vi "NF WF1973_74 sample seq_data.vi"() -> ()   [LabVIEW 2010]
panel:
  in  "Version":dbl=1.0 format="%.2f"
  in  "NEXT?":bool
  in  "Duty 2":dbl=0.01 min=0.01 max=99.99 step=0.01 format="%.2f"
  in  "Phase 2":dbl min=-1800.0 max=1800.0 step=1.0
  in  "Offset 2":dbl min=-10.0 max=10.0 step=1.0 format="%.2f"
  in  "Amplitude 2":dbl min=0.0 max=20.0 step=1.0 format="%.2f"
  in  "Frequency 2":dbl=1e-08 min=1e-08 max=10000000.0 step=0.01 format="%.8f"
  in  "ARB No 2":i16=128
  in  "Duty action 2":u16(ring) items=["Constant", "Keep", "Sweep"]
  in  "Phase action 2":u16(ring) items=["Constant", "Keep", "Sweep"]
  in  "Offset action 2":u16(ring) items=["Constant", "Keep", "Sweep"]
  in  "Amplitude action 2":u16(ring) items=["Constant", "Keep", "Sweep"]
  in  "Frequency action 2":u16(ring) items=["Constant", "Keep", "Sweep"]
  in  "Square Ex(Off) 2":u16(ring) items=["Off", "On"]
  in  "Polarity(Normal) 2":u16(ring) items=["Normal", "Invert"]
  in  "Scale(+/-FS) 2":u16(ring)=1 items=["0/+FS", "+/-FS", "-FS/0"]
  in  "Function(Sin) 2":u16(ring)=2 items=["DC", "Noise", "Sin", "Squ", "USER"]
  in  "Duty":dbl=0.01 min=0.01 max=99.99 step=0.01 format="%.2f"
  in  "Phase":dbl min=-1800.0 max=1800.0 step=1.0
  in  "Offset":dbl min=-10.0 max=10.0 step=1.0 format="%.2f"
  in  "Amplitude":dbl min=0.0 max=20.0 step=1.0 format="%.2f"
  in  "Frequency":dbl=1e-08 min=1e-08 max=10000000.0 step=0.01 format="%.8f"
  in  "ARB No":i16=128
  in  "Duty action":u16(ring) items=["Constant", "Keep", "Sweep"]
  in  "Phase action":u16(ring) items=["Constant", "Keep", "Sweep"]
  in  "Offset action":u16(ring) items=["Constant", "Keep", "Sweep"]
  in  "Amplitude action":u16(ring) items=["Constant", "Keep", "Sweep"]
  in  "Frequency action":u16(ring) items=["Constant", "Keep", "Sweep"]
  in  "Square Ex(Off)":u16(ring) items=["Off", "On"]
  in  "Polarity(Normal)":u16(ring) items=["Normal", "Invert"]
  in  "Scale(+/-FS)":u16(ring)=1 items=["0/+FS", "+/-FS", "-FS/0"]
  in  "Function(Sin)":u16(ring)=2 items=["DC", "Noise", "Sin", "Squ", "USER"]
  in  "Jump count(Infinity)":u16(ring) items=["Infinity", "On"]
  in  "End phase(Off)":u16(ring) items=["Off", "On"]
  in  "Jump step(Off)":u16(ring) items=["Off", "On"]
  in  "Event branch step(Off)":u16(ring) items=["Off", "On"]
  in  "State branch step(Off)":u16(ring) items=["Off", "On"]
  in  "Auto hold(Off)":u16(ring) items=["Off", "On"]
  in  "Parameter(Cont)":u16(ring) items=["Continue", "Stop"]
  in  "End phase":dbl min=0.0 max=360.0 step=1.0
  in  "Jump count":i16=1 min=1 max=999 step=1
  in  "Jump step":i16 min=0 max=255 step=1
  in  "Event branch step":i16 min=0 max=255 step=1
  in  "State branch step":i16 min=0 max=255 step=1
  in  "Step code":i16 min=0 max=15 step=1
  in  "Step time":dbl=0.0001 min=0.0001 max=1000.0 format="%.4f"
  out "Step No":i16
  in  "Trigger polarity(Positive)":u16(ring) items=["Positive", "Negative", "OFF"]
  in  "Digital control(Start)":u16(ring) items=["Start", "State branch"]
  in  "Digital input(Off)":u16(ring) items=["Off", "On"]
  in  "Sync out(Wave)":u16(ring) items=["Wave", "Sequence "]
  in  "Start step(1)":i16=1 min=1 max=255 step=1
  in  "Model(WF1974)":u16(ring)=1 items=["WF1973", "WF1974"]
  out "error out":errorcluster caption="Error OUT"
  in  "error in (no error)":errorcluster caption="Error IN"
  # "Attention!!"
  # "1.Input Model & Version & [Sequence information]\n2.Start VI\n3.Input [Step information] \n4.Input [Channel information] Ch1 & Ch2\n5.Input Parameter\n6.Click to [Next?]\n7.Return to Step 3."
  # "*Firmware version"
  # "This information\n              WF1974 Only!!"
  # "[Ch1 information]"
  # "[Ch2 information]"
  # "[Step information]"
  # "[Sequence information]"
  # "Parameter is \nCont>Next step\nStop>End"
  # "End"
  # "Next step"
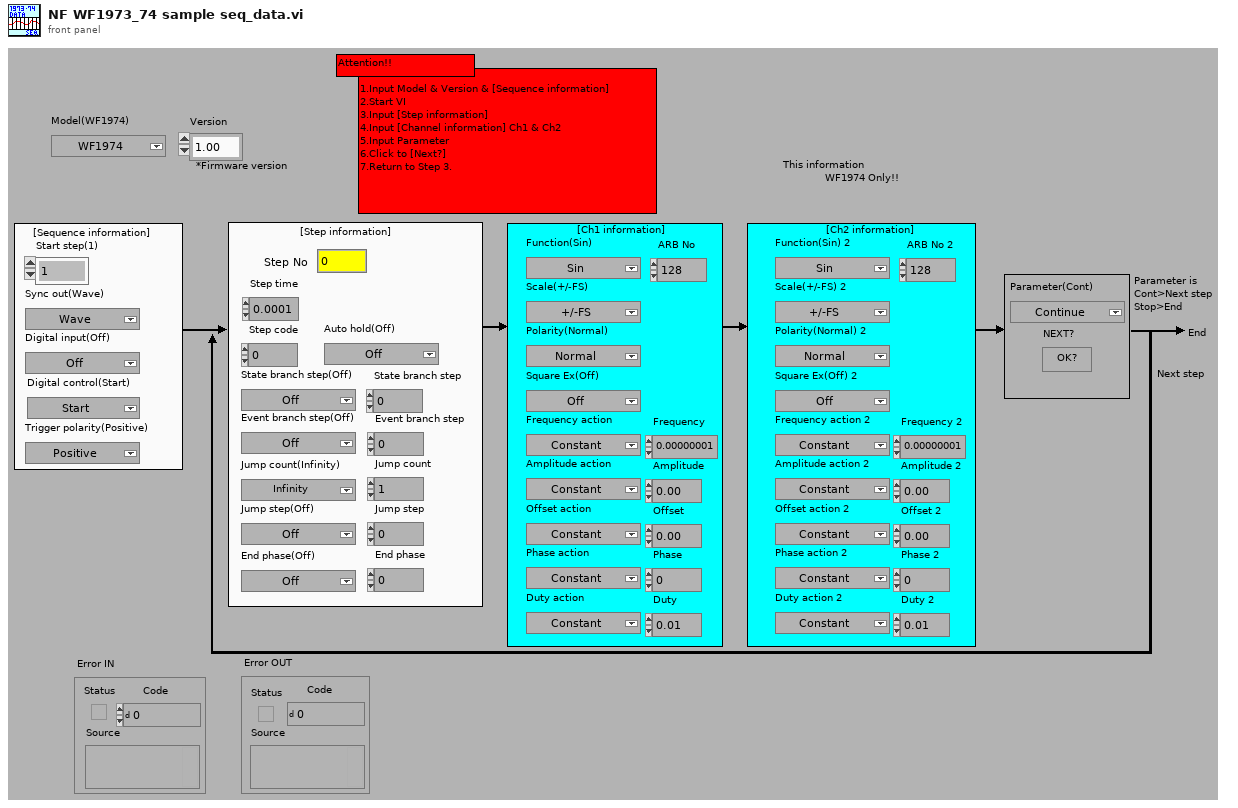
[diagram p1: front panel]
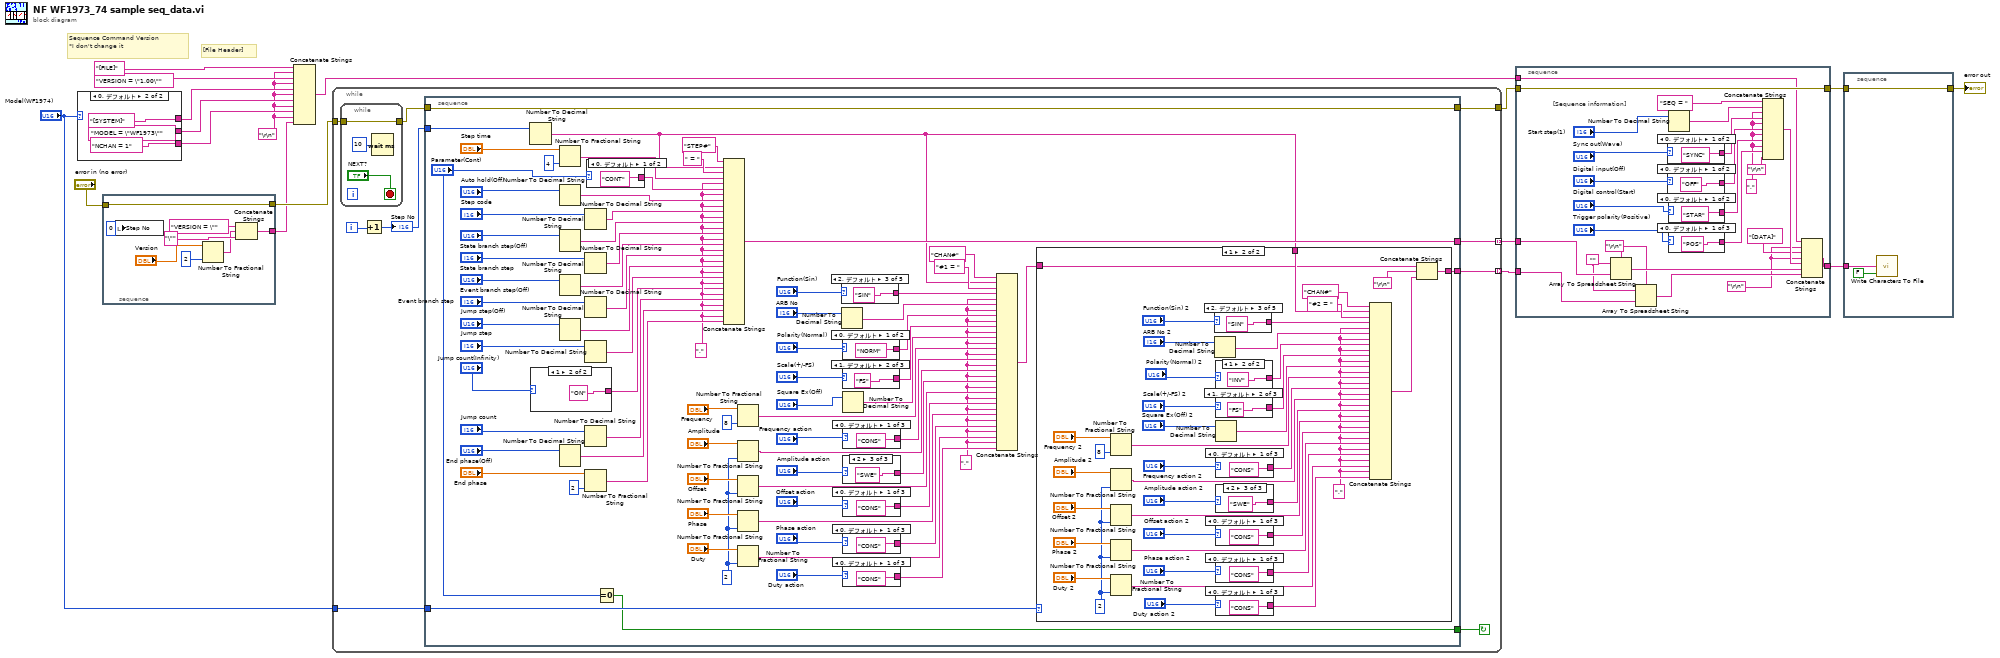
[diagram p0: block diagram]
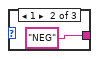
[diagram p2: hidden frame]
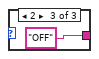
[diagram p3: hidden frame]
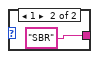
[diagram p4: hidden frame]
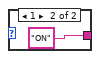
[diagram p5: hidden frame]
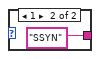
[diagram p6: hidden frame]
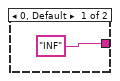
[diagram p7: hidden frame]
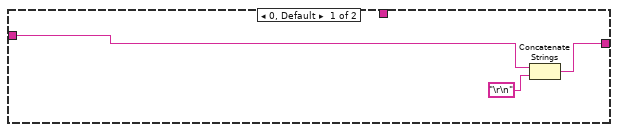
[diagram p8: hidden frame]
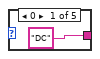
[diagram p9: hidden frame]
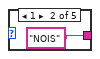
[diagram p10: hidden frame]
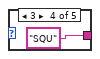
[diagram p11: hidden frame]
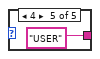
[diagram p12: hidden frame]
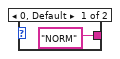
[diagram p13: hidden frame]
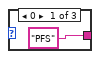
[diagram p14: hidden frame]
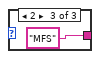
[diagram p15: hidden frame]
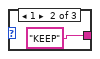
[diagram p16: hidden frame]
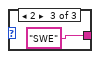
[diagram p17: hidden frame]
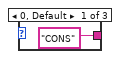
[diagram p18: hidden frame]
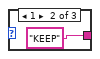
[diagram p19: hidden frame]
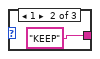
[diagram p20: hidden frame]
diagram:
  w1 = "\r\n"
  # "[File Header]"
  # "Sequence Command Version \n*I don't change it"
  n1 = case shown="0, デフォルト" "Model(WF1974)" {
    tunnel: ["[SYSTEM]" "[SYSTEM]"] -> w7
    tunnel: ["MODEL = \"WF1974\"" "MODEL = \"WF1973\""] -> w6
    tunnel: ["NCHAN = 2" "NCHAN = 1"] -> w5
    frame 1 {
    }
    frame 0, Default {
    }
  }
  n2 = stacked-sequence {
    tunnel: "error in (no error)" -> [w30]
    tunnel: [w30] -> w3
    tunnel: [w25] -> w2
    frame #0 {
      n3 = local write "Step No"(0) -> ()
      n4 = Number To Fractional String(number="Version", precision (6)=i16 2 ("精度 (6)")) -> (F-format string=w27:string)  [unwired: 2 in]
      n5 = Concatenate Strings("VERSION = \"", w27, "\"") -> (w25:string)
    }
  }
  n6 = Concatenate Strings("[FILE]", w1, "VERSION = \"1.00\"", w1, w7, w1, w6, w1, w5, w1, w2) -> (w4:string)
  n7 = while {
    tunnel: [w40] -> w15 mode=indexing
    tunnel: "Model(WF1974)" -> [w39]
    tunnel: [w38] -> w14 mode=indexing
    tunnel: w3 -> [w37]
    tunnel: [w35] -> w13
    i -> [w32]
    stop <- w34 continue-if-true
    n8 = while {
      tunnel: [w215] -> w36
      tunnel: w37 -> [w215]
      stop <- "NEXT?" stop-if-true
      n9 = Wait (ms)(milliseconds to wait=u32 10 ("ミリ秒待ち時間")) -> ()  [unwired: 1 out]
    }
    n10 = Increment(x=w32) -> (x+1=w33:i32)
    "Step No" <- w33
    n11 = stacked-sequence {
      tunnel: [w89] -> w40
      tunnel: w39 -> [w54]
      tunnel: [w52] -> w38
      tunnel: w36 -> [w51]
      tunnel: [w51] -> w35
      tunnel: [w49] -> w34
      tunnel: w33 -> [w47]
      frame #0 {
        w42 = i16 2 ("精度 (6)")
        w45 = ","
        w46 = ","
        n12 = Number To Decimal String(number=w47) -> (decimal integer string=w55:string)  [unwired: 1 in]
        n13 = case shown="1" "Jump count(Infinity)" {
          tunnel: ["INF" "ON"] -> w43
          frame 0, Default {
          }
          frame 1 {
          }
        }
        n14 = Number To Fractional String(number="Step time", precision (6)=i16 4 ("精度 (6)")) -> (F-format string=w102:string)  [unwired: 2 in]
        n15 = Number To Decimal String(number="Auto hold(Off)") -> (decimal integer string=w100:string)  [unwired: 1 in]
        n16 = Number To Decimal String(number="State branch step(Off)") -> (decimal integer string=w98:string)  [unwired: 1 in]
        n17 = Number To Decimal String(number="Event branch step(Off)") -> (decimal integer string=w96:string)  [unwired: 1 in]
        n18 = Number To Decimal String(number="Jump step(Off)") -> (decimal integer string=w94:string)  [unwired: 1 in]
        n19 = Number To Decimal String(number="End phase(Off)") -> (decimal integer string=w91:string)  [unwired: 1 in]
        n20 = Number To Decimal String(number="Step code") -> (decimal integer string=w99:string)  [unwired: 1 in]
        n21 = Number To Decimal String(number="State branch step") -> (decimal integer string=w97:string)  [unwired: 1 in]
        n22 = Number To Decimal String(number="Event branch step") -> (decimal integer string=w95:string)  [unwired: 1 in]
        n23 = Number To Decimal String(number="Jump step") -> (decimal integer string=w93:string)  [unwired: 1 in]
        n24 = Number To Decimal String(number="Jump count") -> (decimal integer string=w92:string)  [unwired: 1 in]
        n25 = Number To Fractional String(number="End phase", precision (6)=i16 2 ("精度 (6)")) -> (F-format string=w90:string)  [unwired: 2 in]
        n26 = case shown="0, デフォルト" "Parameter(Cont)" {
          tunnel: ["CONT" "STOP"] -> w101
          frame 0, Default {
          }
          frame 1 {
          }
        }
        n27 = Equal To 0?(x="Parameter(Cont)") -> (x = 0?=w49:bool)
        n28 = Concatenate Strings("STEP#", w55, " = ", w102, w46, w101, w46, w100, w46, w99, w46, w98, w46, w97, w46, w96, w46, w95, w46, w94, w46, w93, w46, w43, w46, w92, w46, w91, w46, w90) -> (w89:string)
        n29 = Number To Fractional String(number="Frequency", precision (6)=i16 8 ("精度 (6)")) -> (F-format string=w65:string)  [unwired: 2 in]
        n30 = Number To Fractional String(number="Amplitude", precision (6)=w42) -> (F-format string=w63:string)  [unwired: 2 in]
        n31 = Number To Fractional String(number="Offset", precision (6)=w42) -> (F-format string=w61:string)  [unwired: 2 in]
        n32 = Number To Fractional String(number="Phase", precision (6)=w42) -> (F-format string=w59:string)  [unwired: 2 in]
        n33 = Number To Fractional String(number="Duty", precision (6)=w42) -> (F-format string=w57:string)  [unwired: 2 in]
        n34 = case shown="2, デフォルト" "Function(Sin)" {
          tunnel: ["DC" "NOIS" "SIN" "SQU" "USER"] -> w84
          frame 0 {
          }
          frame 1 {
          }
          frame 2, Default {
          }
          frame 3 {
          }
          frame 4 {
          }
        }
        n35 = Number To Decimal String(number="ARB No") -> (decimal integer string=w82:string)  [unwired: 1 in]
        n36 = case shown="0, デフォルト" "Polarity(Normal)" {
          tunnel: ["NORM" "INV"] -> w80
          frame 0, Default {
          }
          frame 1 {
          }
        }
        n37 = case shown="1, デフォルト" "Scale(+/-FS)" {
          tunnel: ["PFS" "FS" "MFS"] -> w77
          frame 0 {
          }
          frame 1, Default {
          }
          frame 2 {
          }
        }
        n38 = Number To Decimal String(number="Square Ex(Off)") -> (decimal integer string=w76:string)  [unwired: 1 in]
        n39 = case shown="0, デフォルト" "Frequency action" {
          tunnel: ["CONS" "KEEP" "SWE"] -> w64
          frame 0, Default {
          }
          frame 1 {
          }
          frame 2 {
          }
        }
        n40 = case shown="2" "Amplitude action" {
          tunnel: ["CONS" "KEEP" "SWE"] -> w62
          frame 0, Default {
          }
          frame 1 {
          }
          frame 2 {
          }
        }
        n41 = case shown="0, デフォルト" "Offset action" {
          tunnel: ["CONS" "KEEP" "SWE"] -> w60
          frame 0, Default {
          }
          frame 1 {
          }
          frame 2 {
          }
        }
        n42 = case shown="0, デフォルト" "Phase action" {
          tunnel: ["CONS" "KEEP" "SWE"] -> w58
          frame 0, Default {
          }
          frame 1 {
          }
          frame 2 {
          }
        }
        n43 = case shown="0, デフォルト" "Duty action" {
          tunnel: ["CONS" "KEEP" "SWE"] -> w56
          frame 0, Default {
          }
          frame 1 {
          }
          frame 2 {
          }
        }
        n44 = Concatenate Strings("CHAN#", w55, "#1 = ", w84, w45, w82, w45, w80, w45, w77, w45, w76, w45, w65, w45, w64, w45, w63, w45, w62, w45, w61, w45, w60, w45, w59, w45, w58, w45, w57, w45, w56) -> (w53:string)
        n45 = case shown="1" w54 {
          tunnel: w55 -> [_ w131]
          tunnel: w53 -> [w120 w129]
          tunnel: [w121 w130] -> w52
          frame 0, Default {
            n46 = Concatenate Strings(w120, "\r\n") -> (w121:string)
          }
          frame 1 {
            w125 = ","
            w123 = i16 2 ("精度 (6)")
            n47 = Number To Fractional String(number="Frequency 2", precision (6)=i16 8 ("精度 (6)")) -> (F-format string=w152:string)  [unwired: 2 in]
            n48 = Number To Fractional String(number="Amplitude 2", precision (6)=w123) -> (F-format string=w154:string)  [unwired: 2 in]
            n49 = Number To Fractional String(number="Offset 2", precision (6)=w123) -> (F-format string=w156:string)  [unwired: 2 in]
            n50 = Number To Fractional String(number="Phase 2", precision (6)=w123) -> (F-format string=w158:string)  [unwired: 2 in]
            n51 = Number To Fractional String(number="Duty 2", precision (6)=w123) -> (F-format string=w160:string)  [unwired: 2 in]
            n52 = case shown="2, デフォルト" "Function(Sin) 2" {
              tunnel: ["DC" "NOIS" "SIN" "SQU" "USER"] -> w147
              frame 0 {
              }
              frame 1 {
              }
              frame 2, Default {
              }
              frame 3 {
              }
              frame 4 {
              }
            }
            n53 = Number To Decimal String(number="ARB No 2") -> (decimal integer string=w148:string)  [unwired: 1 in]
            n54 = case shown="1" "Polarity(Normal) 2" {
              tunnel: ["NORM" "INV"] -> w149
              frame 0, Default {
              }
              frame 1 {
              }
            }
            n55 = case shown="1, デフォルト" "Scale(+/-FS) 2" {
              tunnel: ["PFS" "FS" "MFS"] -> w150
              frame 0 {
              }
              frame 1, Default {
              }
              frame 2 {
              }
            }
            n56 = Number To Decimal String(number="Square Ex(Off) 2") -> (decimal integer string=w151:string)  [unwired: 1 in]
            n57 = case shown="0, デフォルト" "Frequency action 2" {
              tunnel: ["CONS" "KEEP" "SWE"] -> w153
              frame 0, Default {
              }
              frame 1 {
              }
              frame 2 {
              }
            }
            n58 = case shown="2" "Amplitude action 2" {
              tunnel: ["CONS" "KEEP" "SWE"] -> w155
              frame 0, Default {
              }
              frame 1 {
              }
              frame 2 {
              }
            }
            n59 = case shown="0, デフォルト" "Offset action 2" {
              tunnel: ["CONS" "KEEP" "SWE"] -> w157
              frame 0, Default {
              }
              frame 1 {
              }
              frame 2 {
              }
            }
            n60 = case shown="0, デフォルト" "Phase action 2" {
              tunnel: ["CONS" "KEEP" "SWE"] -> w159
              frame 0, Default {
              }
              frame 1 {
              }
              frame 2 {
              }
            }
            n61 = case shown="0, デフォルト" "Duty action 2" {
              tunnel: ["CONS" "KEEP" "SWE"] -> w161
              frame 0, Default {
              }
              frame 1 {
              }
              frame 2 {
              }
            }
            n62 = Concatenate Strings("CHAN#", w131, "#2 = ", w147, w125, w148, w125, w149, w125, w150, w125, w151, w125, w152, w125, w153, w125, w154, w125, w155, w125, w156, w125, w157, w125, w158, w125, w159, w125, w160, w125, w161) -> (w126:string)
            n63 = Concatenate Strings(w129, "\r\n", w126) -> (w130:string)
          }
        }
      }
    }
  }
  n64 = stacked-sequence {
    tunnel: w15 -> [w222]
    tunnel: w14 -> [w220]
    tunnel: [w228] -> w12
    tunnel: [w227] -> w11
    tunnel: w13 -> [w227]
    tunnel: w4 -> [w225]
    frame #0 {
      w217 = "\r\n"
      w218 = "\r\n"
      w221 = ""
      w230 = ","
      # "[Sequence information]"
      n65 = Array To Spreadsheet String(delimiter (Tab)=w218, array=w222, 3:w221) -> (spreadsheet string=w226:string)
      n66 = Array To Spreadsheet String(delimiter (Tab)=w218, array=w220, 3:w221) -> (spreadsheet string=w219:string)
      n67 = case shown="0, デフォルト" "Sync out(Wave)" {
        tunnel: ["SYNC" "SSYN"] -> w234
        frame 0, Default {
        }
        frame 1 {
        }
      }
      n68 = case shown="0, デフォルト" "Digital input(Off)" {
        tunnel: ["OFF" "ON"] -> w233
        frame 0, Default {
        }
        frame 1 {
        }
      }
      n69 = Number To Decimal String(number="Start step(1)") -> (decimal integer string=w235:string)  [unwired: 1 in]
      n70 = case shown="0, デフォルト" "Digital control(Start)" {
        tunnel: ["STAR" "SBR"] -> w232
        frame 0, Default {
        }
        frame 1 {
        }
      }
      n71 = case shown="0, デフォルト" "Trigger polarity(Positive)" {
        tunnel: ["POS" "NEG" "OFF"] -> w231
        frame 0, Default {
        }
        frame 1 {
        }
        frame 2 {
        }
      }
      n72 = Concatenate Strings("SEQ = ", w235, w230, w234, w230, w233, w230, w232, w230, w231, "\r\n") -> (w224:string)
      n73 = Concatenate Strings(w225, w217, "[DATA]", w217, w224, w226, w219) -> (w228:string)
    }
  }
  n74 = stacked-sequence {
    tunnel: w12 -> [w253]
    tunnel: [w251] -> w10
    tunnel: w11 -> [w251]
    frame #0 {
      n75 = call <vilib>:"Write Characters To File.vi"("append to file? (new file:F)"=FALSE, "character string"=w253) -> ()  [unwired: 3 in, 1 out]
    }
  }
  "error out" <- w10
